vi "Set SysCfg Session.vi"(8 "error in (no error)":errorcluster, 10 "SysCfg Session":refnum<k21>, 11 "RT Management Session in":refnum<class "RT Management.lvclass">) -> (0 "error out":errorcluster, 3 "RT Management Session out":refnum<class "RT Management.lvclass">)   [LabVIEW 2015, in "RT Management.lvlib" / "RT Management.lvclass"]
uses:
  RT Management.lvclass
  RT Management.lvclass/RT Management.ctl
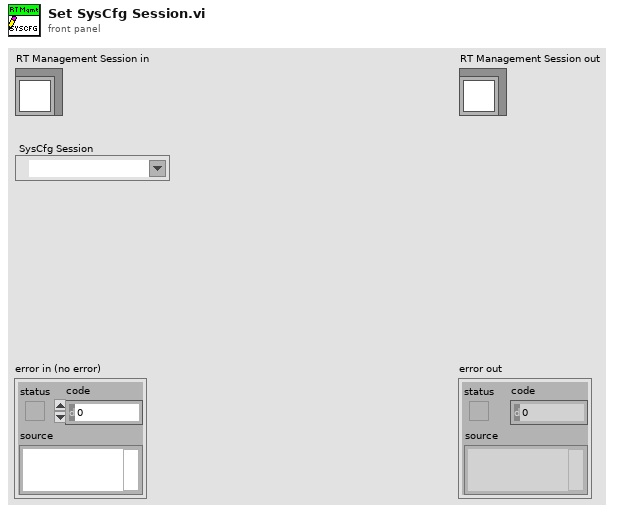
[diagram p1: front panel]
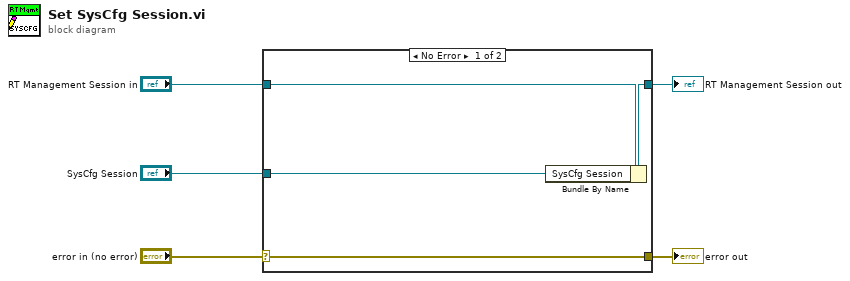
[diagram p0: block diagram]
diagram:
  n1 = case shown="No Error" "error in (no error)" {
    selector: "error in (no error)" -> [w9 w10]
    tunnel: [w9 w10] -> w4
    tunnel: [w7 w11] -> w2
    tunnel: "RT Management Session in" -> [w8 w11]
    tunnel: "SysCfg Session" -> [w6 _]
    frame No Error {
      n2 = Bundle By Name(cluster=w8, "SysCfg Session"=w6) -> (w7:refnum<class "RT Management.lvclass">)
    }
    frame Error {
    }
  }
  "error out" <- w4
  "RT Management Session out" <- w2
